vi "GiegerInput.vi"() -> ()   [LabVIEW 2014]
uses:
  <vilib>/platform/TimedLoop/XDataNode/XDataNode.xnode
  <vilib>/Platform/TimedLoop/XDataNode/nitl_modes.ctl
  <vilib>/Platform/TimedLoop/XDataNode/XDNodeRunTimeDep.lvlib
  <vilib>/Platform/TimedLoop/XDataNode/wakeup.ctl
  <vilib>/Platform/TimedLoop/XDataNode/timing_clust.ctl
  <vilib>/Utility/file.llb/Write To Spreadsheet File (DBL).vi
panel:
  out "x+y":dbl[](array[numeric])
  in  "Aquisition Time (s)":i64
  out "Waveform Graph":waveform(dbl)(graph)
  in  "input cluster":T1
  in  "File to save":path=path "C:/Users/zchmlk/Desktop/week7/GainData.txt"
  out "Error":errorcluster
  in  "Period (s)":i64=1000
  in  "?":bool
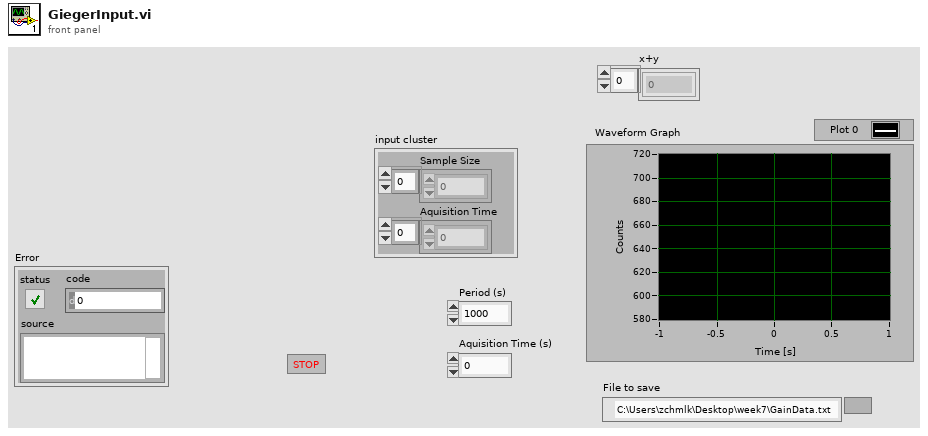
[diagram p1: front panel]
types:
  T1 = cluster{"Sample Size":i16[], "Aquisition Time":dbl[]}
  T2 = typedef "XDNodeRunTimeDep.lvlib/timing_clust.ctl" = cluster{"Expected End [f-1]":u64, "Actual End [f-1]":u64, "Finished Late? [f-1]":bool, "Expected End [i-1]":u64, "Actual End [i-1]":u64, "Finished Late? [i-1]":bool, "Expected Start [i]":u64, "Actual Start [i]":u64, "Expected Start [f]":u64, "Actual Start [f]":u64, "Source Name":string, "Structure Name":string, "Period":i64, "Deadline":i64, "Offset":i64, "Start":i64, "Priority":i32, "Timeout":i32, "Mode":T3, "Wakeup Reason":T4, "Error":errorcluster, "Source Type":string, "Secondary Source Type":string, "Global End Time":u64, "Global Start Time":u64, "Frame Duration":u64, "Iteration Duration":u64, "Assigned CPU":i32, "I/O Scan Engine Mode":u32}
  T3 = typedef "XDNodeRunTimeDep.lvlib/nitl_modes.ctl" = enum32{"No Change", "Process missed periods, maintain original phase", "Discard missed periods, maintain original phase", "Process missed periods, ignore original phase", "Discard missed periods, ignore original phase"}
  T4 = typedef "XDNodeRunTimeDep.lvlib/wakeup.ctl" = enum32{"Normal", "Aborted", "Asynchronous wakeup", "Timing source error", "Timed loop error", "Timeout"}
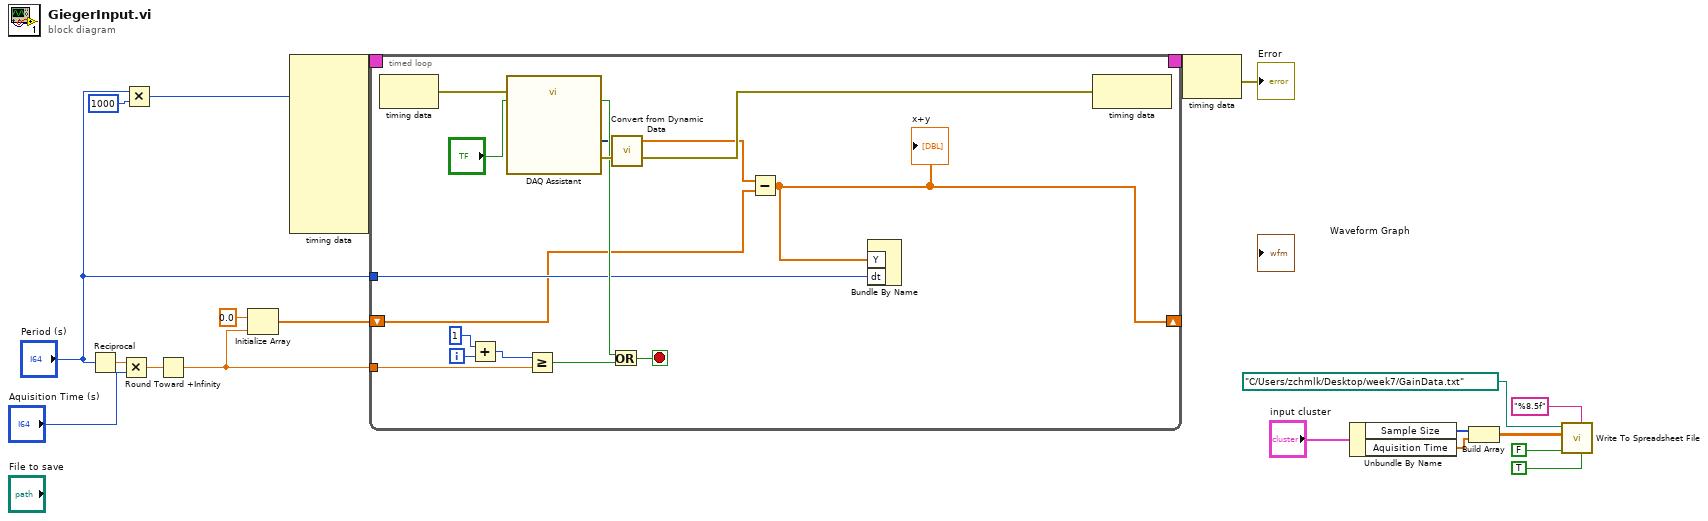
[diagram p0: block diagram]
diagram:
  n1 = Reciprocal(x="Period (s)") -> (1/x=w7:dbl)
  n2 = Multiply(x=w7, y="Aquisition Time (s)") -> (x*y=w2:dbl)
  n3 = Multiply(x="Period (s)", y=1000) -> (x*y=w8:i64)
  n4 = Round Toward +Infinity(x=w2) -> (ceil(x): smallest int >= x=w1:dbl)
  n5 = Initialize Array(0.0, w1) -> (w4:dbl[])
  n6 = node-c288(w8) -> (w20:T2)  [unwired: 9 in]
  n7 = timed-loop {
    timing: w20 -> [_]
    timing-out: [_] -> w19
    shift-right: [w21] -> _
    shift-left: w4 -> [w22]
    tunnel: w1 -> [w33]
    tunnel: "Period (s)" -> [w24]
    i -> [w28]
    stop <- w32 stop-if-true
    n8 = node-c288() -> (w35:errorcluster)  [unwired: 1 in]
    n9 = Add(x=1, y=w28) -> (x+y=w27:i32)
    n10 = call "DAQ Assistant"("error in"=w35, "stop (F)"="?") -> ("data"=w26:dynamicdata, "stopped"=w30:bool, "error out"=w36:errorcluster)  [unwired: 14 in, 1 out]
    n11 = Greater Or Equal?(x=w27, y=w33) -> (x >= y?=w31:bool)
    n12 = Or(x=w30, y=w31) -> (x .or. y?=w32:bool)
    n13 = call "Convert from Dynamic Data"("Dynamic Data Type"=w26) -> ("Array"=w23:dbl[])  [unwired: 3 in]
    n14 = Subtract(x=w23, y=w22) -> (x-y=w21:dbl[])
    "x+y" <- w21
    n15 = Bundle By Name("Y"=w21, "dt"=w24) -> (w25:waveform(dbl))  [unwired: 1 in]
    n16 = node-c288(w36) -> ()  [unwired: 1 out]
  }
  n17 = node-c288(w19) -> (→"Error":errorcluster)
  n18 = Unbundle By Name("input cluster") -> ("Sample Size"=w15:i16[], "Aquisition Time"=w14:dbl[])
  n19 = Build Array(w15, w14) -> (w11:dbl[][])
  n20 = call-poly <vilib>:"Write To Spreadsheet File.vi"("transpose? (no:F)"=TRUE, "format (%.3f)"="%8.5f", "append to file? (new file:F)"=FALSE, "2D data"=w11, "file path (dialog if empty)"=path "C:/Users/zchmlk/Desktop/week7/GainData.txt") -> ()  [unwired: 3 in, 1 out]
